vi "Settings Dialog.vi"(8 "error in (no error)":errorcluster, 11 "Settings in":T3={"Logging Configuration"={"Log File Base Path"=path "", "NbrIma"=1}, "camera"={"Camera.lvclass"=refnum, "InClusTiming 2"={"Pixelclock"=24, "Exposure"=46.39115, "ExposureTimeBase"=2, "Framerate"=14.99615, "TriggerMode"=0}, "ROI"={"PosX"=0, "PosY"=0, "Width"=0, "Height"=0}, "File Path Control"=path "", "mirror.lvclass"=refnum}} {"camera"."InClusTiming 2"."TriggerMode" items=["Auto", "Software", "External sequence start ", "External exposure control"]; "camera"."InClusTiming 2"."ExposureTimeBase" items=["nanoseconds", "microseconds", "milliseconds"]; "camera"."InClusTiming 2"."Pixelclock" min=1 max=400 step=1 scale=0.05915..400.0 scale format="%#.3g"; "camera"."InClusTiming 2"."Framerate" min=0.05915 max=2000.0 step=1.0 scale=0.05915..100.0 scale format="%#.3g"; "camera"."InClusTiming 2"."Exposure" min=0.05915 max=2000.0 step=1.0 scale=0.05915..100.0 scale format="%#.3g"; "Logging Configuration"."NbrIma" min=1 step=1}) -> (0 "error out":errorcluster, 1 "Cancelled?":bool, 2 "UI Refresh Needed?":bool, 3 "Settings out":T3={"Logging Configuration"={"Log File Base Path"=path "F:/DATA/test.fits", "NbrIma"=1}, "camera"={"Camera.lvclass"=refnum, "InClusTiming 2"={"Pixelclock"=24, "Exposure"=46.39115, "ExposureTimeBase"=2, "Framerate"=14.99615, "TriggerMode"=0}, "ROI"={"PosX"=0, "PosY"=0, "Width"=0, "Height"=0}, "File Path Control"=path "", "mirror.lvclass"=refnum}} {"camera"."InClusTiming 2"."TriggerMode" items=["Auto", "Software", "External sequence start ", "External exposure control"]; "camera"."InClusTiming 2"."ExposureTimeBase" items=["nanoseconds", "microseconds", "milliseconds"]; "camera"."InClusTiming 2"."Pixelclock" min=1 max=400 step=1 scale=0.05915..400.0 scale format="%#.3g"; "camera"."InClusTiming 2"."Framerate" min=0.05915 max=2000.0 step=1.0 scale=0.05915..100.0 scale format="%#.3g"; "camera"."InClusTiming 2"."Exposure" min=0.05915 max=2000.0 step=1.0 scale=0.05915..100.0 scale format="%#.3g"; "Logging Configuration"."NbrIma" min=1 step=1})   [LabVIEW 2020, in "Settings.lvlib"]
doc: "Dialog for selecting user specified settings."
uses:
  Settings.lvlib
  Settings.ctl
  CLASS/Image Acquisition Class/Camera.lvclass
  MIRROR/mirror.lvclass
  LOGGING/Logging Configuration.ctl
  ACQUISITION/HardwareConfiguration.ctl
  <vilib>/Utility/xml.llb/Read From XML File(string).vi
  <vilib>/Utility/xml.llb/Write to XML File(string).vi
  LOGGING/Logging.lvlib
  ACQUISITION/Acquisition.lvlib
panel:
  in  "InClusTiming 2":T1={"Pixelclock"=24, "Exposure"=14.99615, "ExposureTimeBase"=2, "Framerate"=14.99615, "TriggerMode"=0} {"TriggerMode" items=["Auto", "Software", "External sequence start ", "External exposure control"]; "ExposureTimeBase" items=["nanoseconds", "microseconds", "milliseconds"]; "Pixelclock" min=1 max=400 step=1 scale=0.05915..400.0 scale format="%#.3g"; "Framerate" min=0.05915 max=2000.0 step=1.0 scale=0.05915..100.0 scale format="%#.3g"; "Exposure" min=0.05915 max=2000.0 step=1.0 scale=0.05915..100.0 scale format="%#.3g"}
  in  "ROI":T2={"PosX"=0, "PosY"=0, "Width"=304, "Height"=304}
  in  "File Path Control":path=path "F:/TECHNIQUE/ROLLMOPS/DISTRIB_ROLLMOPS_CLOVIS_OA/lib_LV/CAMERA/IDS/Param iDS/paramCamera_20190715_test.ini"
  in  "NbrIma":i32=32 min=1 step=1
  in  "Log File Path":path=path "F:/DATA/toto.FITS"
  in  "Cancel Button":bool
  in  "OK Button":bool
  # "Non visible portion of dialog (needed for connector pane)."
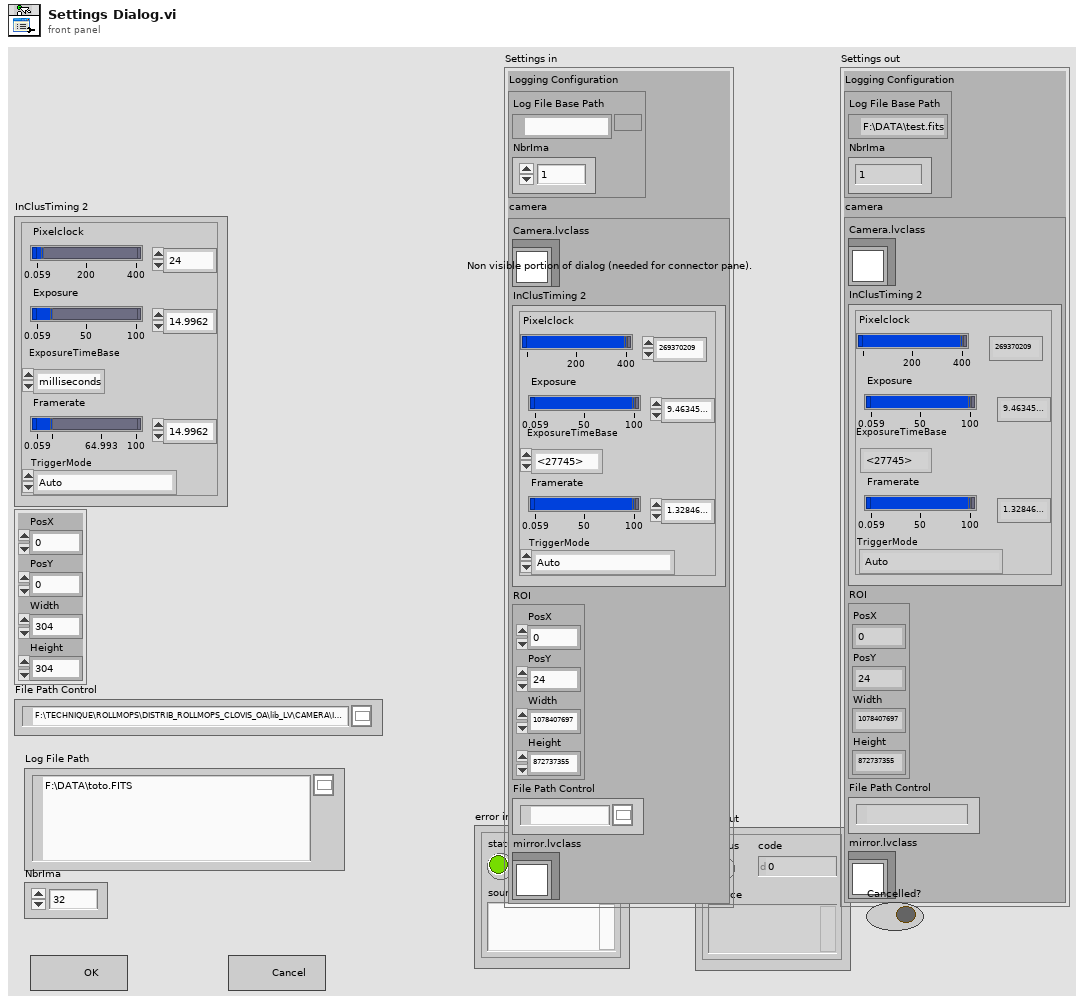
[diagram p1: front panel]
types:
  T1 = cluster{"Pixelclock":i32, "Exposure":dbl, "ExposureTimeBase":u16, "Framerate":dbl, "TriggerMode":u16}
  T2 = cluster{"PosX":i32, "PosY":i32, "Width":i32, "Height":i32}
  T3 = typedef "Settings.lvlib/Settings.ctl" = cluster{"Logging Configuration":T4, "camera":T5}
  T4 = typedef "Logging.lvlib/Logging Configuration.ctl" = cluster{"Log File Base Path":path, "NbrIma":i32}
  T5 = typedef "Acquisition.lvlib/HardwareConfiguration.ctl" = cluster{"Camera.lvclass":refnum<class "Camera.lvclass">, "InClusTiming 2":cluster{"Pixelclock":i32, "Exposure":dbl, "ExposureTimeBase":u16, "Framerate":dbl, "TriggerMode":u16}, "ROI":cluster{"PosX":i32, "PosY":i32, "Width":i32, "Height":i32}, "File Path Control":path, "mirror.lvclass":refnum<class "mirror.lvclass">}
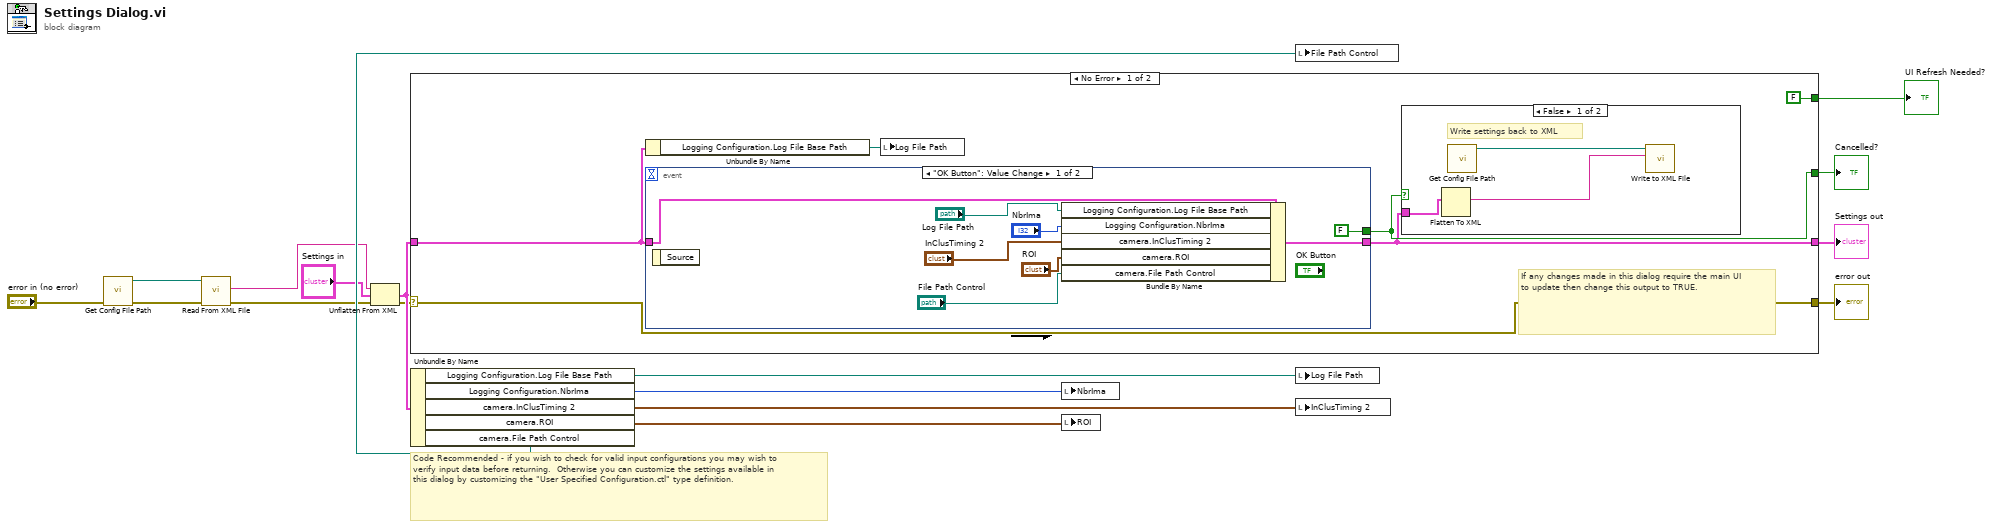
[diagram p0: block diagram]
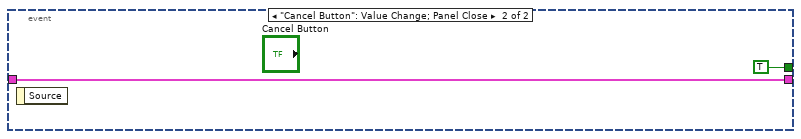
[diagram p3: hidden frame]
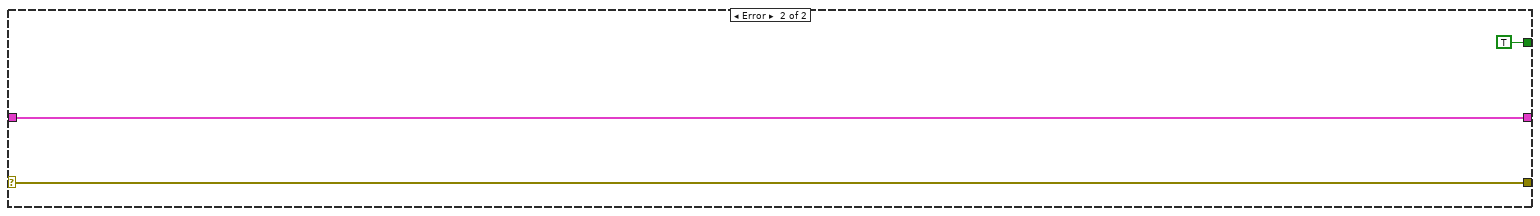
[diagram p4: hidden frame]
diagram:
  # "Code Recommended - if you wish to check for valid input configurations you may wish to verify input data before returning.  Otherwise you can customize the settings available in this dialog by customizing the \"User Specified Configuration.ctl\" type definition."
  n1 = call "Get Config File Path.vi"("error in (no error)"="error in (no error)") -> ("error out"=w4:errorcluster, "XML File Path"=w5:path)  [unwired: 9 in]
  n2 = call-poly <vilib>:"Read From XML File.vi"("error in (no error)"=w4, "XML File Path"=w5) -> ("error out"=w3:errorcluster, "XML Elements"=w8:string)  [unwired: 7 in, 1 out]
  n3 = Unflatten From XML(xml string=w8, type="Settings in", error in (no error)=w3) -> (value=w6:T3, error out=w1:errorcluster)
  n4 = case shown="No Error" w1 {
    selector: w1 -> [w23 w39]
    tunnel: [w23 w39] -> w17
    tunnel: w6 -> [w19 w38]
    tunnel: [w20 w38] -> w16
    tunnel: [FALSE ("UI Refresh Needed?") _] -> w15
    tunnel: [w21 TRUE ("UI Refresh Needed?")] -> w14
    frame No Error {
      # "If any changes made in this dialog require the main UI to update then change this output to TRUE."
      n5 = Unbundle By Name(w19) -> ("Logging Configuration.Log File Base Path"=w18:path)
      n6 = event shown="[0] \"OK Button\": Value Change" {
        selector: _ -> [_ _]
        dyn-events: _ -> [_ _]
        timeout: _ -> [_ _]
        tunnel: [w32 w36] -> w20
        tunnel: w19 -> [w33 w36]
        tunnel: [FALSE ("UI Refresh Needed?") TRUE ("UI Refresh Needed?")] -> w21
        event "OK Button": Value Change {
          n7 = event-data() -> ()  [unwired: 1 in, 1 out]
          n8 = Bundle By Name(cluster=w33, "Logging Configuration.Log File Base Path"="Log File Path", "Logging Configuration.NbrIma"="NbrIma", "camera.InClusTiming 2"="InClusTiming 2", "camera.ROI"="ROI", "camera.File Path Control"="File Path Control") -> (w32:T3)
        }
        event "Cancel Button": Value Change; Panel Close {
          n9 = event-data() -> ()  [unwired: 1 in, 1 out]
        }
      }
      n10 = local write "Log File Path"(w18) -> ()
      n11 = case shown="False" w21 {
        tunnel: w20 -> [w25 _]
        frame False {
          # "Write settings back to XML"
          n12 = Flatten To XML(6:w25) -> (2:w24:string)
          n13 = call "Get Config File Path.vi"() -> ("XML File Path"=w26:path)  [unwired: 10 in, 1 out]
          n14 = call-poly <vilib>:"Write to XML File.vi"("XML Input"=w24, "XML File Path"=w26) -> ()  [unwired: 7 in, 3 out]
        }
        frame True {
        }
      }
    }
    frame Error {
    }
  }
  "UI Refresh Needed?" <- w15
  "error out" <- w17
  "Settings out" <- w16
  "Cancelled?" <- w14
  n15 = Unbundle By Name(w6) -> ("Logging Configuration.Log File Base Path"=w10:path, "Logging Configuration.NbrIma"=w9:i32, "camera.InClusTiming 2"=w13:T1, "camera.ROI"=w12:T2, "camera.File Path Control"=w11:path)
  n16 = local write "NbrIma"(w9) -> ()
  n17 = local write "ROI"(w12) -> ()
  n18 = local write "File Path Control"(w11) -> ()
  n19 = local write "Log File Path"(w10) -> ()
  n20 = local write "InClusTiming 2"(w13) -> ()
